vi "Lin_Rohner_lab1_ex1.vi"() -> ()   [LabVIEW 2019]
uses:
  <vilib>/Platform/TimedLoop/XDataNode/timing_clust.ctl
  <vilib>/Platform/TimedLoop/XDataNode/nitl_modes.ctl
  <vilib>/Platform/TimedLoop/XDataNode/wakeup.ctl
  <vilib>/Analysis/baseanly.llb/Mean (DBL).vi
  <vilib>/platform/TimedLoop/XDataNode/XDataNode.xnode
  <vilib>/Platform/TimedLoop/XDataNode/XDNodeRunTimeDep.lvlib
  <vilib>/Analysis/NI_AALBase.lvlib
panel:
  in  "Acceleration unit":bool
  out "min value":dbl
  out "max value":dbl
  out "mean":dbl format="%0.2f"
  out "Current Value":dbl
  in  "Channel select":tag
  in  "READY":bool
  out "Entire Acceleration Signal-Plot":dynamicdata(graph)
  out "Live Acceleration Signal":dbl(graph)
  in  "STOP":bool
  out "Current Data Point":dbl
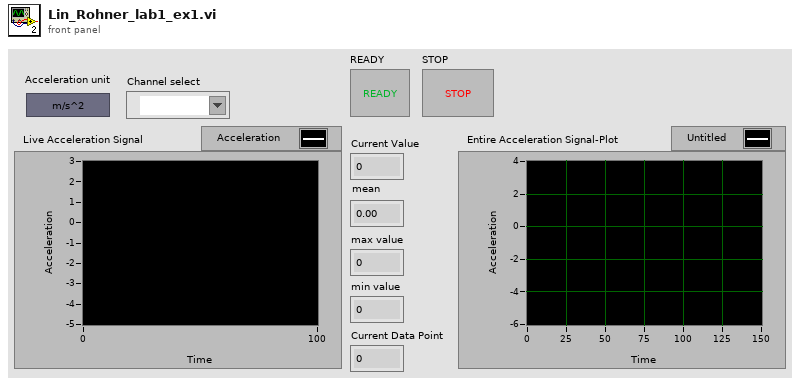
[diagram p1: front panel]
types:
  T1 = typedef "XDNodeRunTimeDep.lvlib/timing_clust.ctl" = cluster{"Expected End [f-1]":u64, "Actual End [f-1]":u64, "Finished Late? [f-1]":bool, "Expected End [i-1]":u64, "Actual End [i-1]":u64, "Finished Late? [i-1]":bool, "Expected Start [i]":u64, "Actual Start [i]":u64, "Expected Start [f]":u64, "Actual Start [f]":u64, "Source Name":string, "Structure Name":string, "Period":i64, "Deadline":i64, "Offset":i64, "Start":i64, "Priority":i32, "Timeout":i32, "Mode":T2, "Wakeup Reason":T3, "Error":errorcluster, "Source Type":string, "Secondary Source Type":string, "Global End Time":u64, "Global Start Time":u64, "Frame Duration":u64, "Iteration Duration":u64, "Assigned CPU":i32, "I/O Scan Engine Mode":u32}
  T2 = typedef "XDNodeRunTimeDep.lvlib/nitl_modes.ctl" = enum32{"No Change", "Process missed periods, maintain original phase", "Discard missed periods, maintain original phase", "Process missed periods, ignore original phase", "Discard missed periods, ignore original phase"}
  T3 = typedef "XDNodeRunTimeDep.lvlib/wakeup.ctl" = enum32{"Normal", "Aborted", "Asynchronous wakeup", "Timing source error", "Timed loop error", "Timeout"}
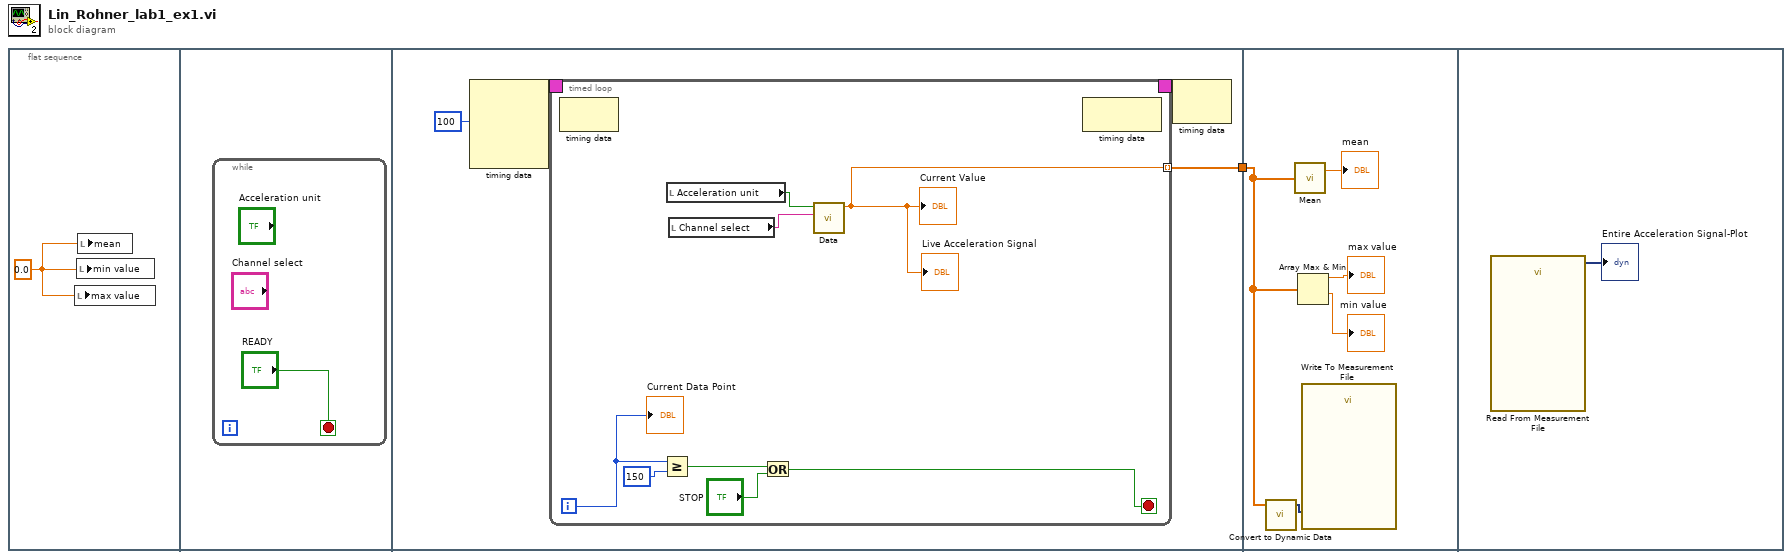
[diagram p0: block diagram]
diagram:
  n1 = flat-sequence {
    tunnel: [w4] -> w1
    tunnel: w1 -> [w23]
    frame #0 {
      w2 = 0.0 ("mean")
      n2 = local write "max value"(w2) -> ()
      n3 = local write "min value"(w2) -> ()
      n4 = local write "mean"(w2) -> ()
    }
    frame #1 {
      n5 = while {
        stop <- "READY" stop-if-true
      }
    }
    frame #2 {
      n6 = node-c288(i64 100 ("Period")) -> (w7:T1)  [unwired: 3 in]
      n7 = timed-loop {
        timing: w7 -> [_]
        timing-out: [_] -> w6
        tunnel: [w8] -> w4 mode=indexing
        i -> [w15]
        stop <- w11 stop-if-true
        n8 = node-c288() -> ()  [unwired: 1 in, 1 out]
        n9 = Greater Or Equal?(x=w15, y=150) -> (x >= y?=w13:bool)
        n10 = local read "Acceleration unit"() -> (w10:bool)
        n11 = local read "Channel select"() -> (w9:tag)
        n12 = Or(x=w13, y="STOP") -> (x .or. y?=w11:bool)
        n13 = call "Data.vi"("Channel select"=w9, "Acceleration in\nm/s^2    or    g"=w10) -> ("Data"=w8:dbl)  [unwired: 9 in]
        "Live Acceleration Signal" <- w8
        "Current Value" <- w8
        n14 = node-c288() -> ()  [unwired: 1 in, 1 out]
        "Current Data Point" <- w15
      }
      n15 = node-c288(w6) -> ()  [unwired: 1 out]
    }
    frame #3 {
      n16 = call "Convert to Dynamic Data"("Array"=w23) -> ("Dynamic Data Type"=w22:dynamicdata)  [unwired: 3 in]
      n17 = call-poly <vilib>:"Mean.vi"("X"=w23) -> ("mean"=→"mean":dbl)  [unwired: 1 out]
      n18 = Array Max & Min(array=w23) -> (max value=→"max value":dbl, min value=→"min value":dbl)  [unwired: 2 out]
      n19 = call "Write To Measurement File"("Signals"=w22) -> ()  [unwired: 16 in, 3 out]
    }
    frame #4 {
      n20 = call "Read From Measurement File"() -> ("Signals"=→"Entire Acceleration Signal-Plot":dynamicdata)  [unwired: 6 in, 5 out]
    }
  }
